vi "ep_Check Error (N CH).vi"(0 "spectra information":T1, 5 "slip":dbl[](array[numeric]), 7 "max sideband order (10)":u8=10, 9 "fundamental frequency [Hz]":dbl, 11 "error in (no error)":errorcluster) -> (4 "dup spectra information":T1, 6 "dup slip":dbl[](array[numeric]), 10 "dup fundamental frequency [Hz]":dbl, 15 "error out":errorcluster)   [LabVIEW 2014, in "NI_EP_Motor Monitoring.lvlib"]
uses:
  <vilib>/addons/Electrical Power/Motor Monitoring/NI_EP_Motor Monitoring.lvlib
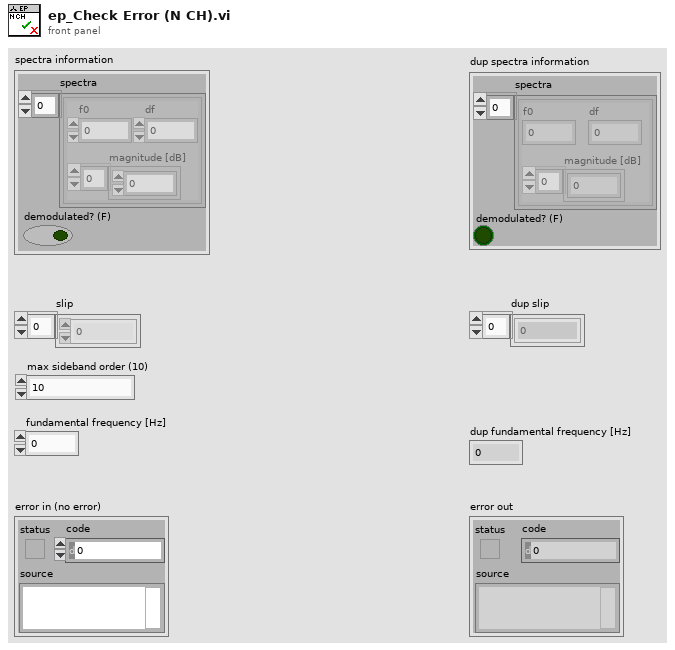
[diagram p1: front panel]
types:
  T1 = cluster{"spectra":cluster{"f0":dbl, "df":dbl, "magnitude [dB]":dbl[]}[], "demodulated? (F)":bool}
  T2 = cluster{"f0":dbl, "df":dbl, "magnitude [dB]":dbl[]}[]
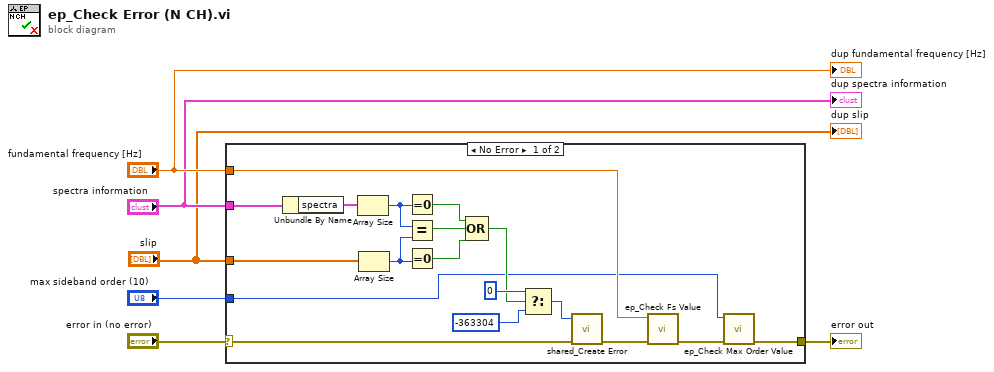
[diagram p0: block diagram]
diagram:
  n1 = case shown="No Error" "error in (no error)" {
    selector: "error in (no error)" -> [w19 w25]
    tunnel: "spectra information" -> [w21 _]
    tunnel: "slip" -> [w10 _]
    tunnel: "fundamental frequency [Hz]" -> [w11 _]
    tunnel: [w8 w25] -> w5
    tunnel: "max sideband order (10)" -> [w7 _]
    frame No Error {
      n2 = Unbundle By Name(w21) -> ("spectra"=w20:T2)
      n3 = Array Size(array=w20) -> (size(s)=w12:i32)
      n4 = Array Size(array=w10) -> (size(s)=w17:i32)
      n5 = Equal To 0?(x=w12) -> (x = 0?=w16:bool)
      n6 = Equal?(x=w12, y=w17) -> (x = y?=w15:bool)
      n7 = Equal To 0?(x=w17) -> (x = 0?=w14:bool)
      n8 = Compound Arithmetic op=OR(w16, w15, w14) -> (w13:bool)
      n9 = Select(t=0 ("error code (0)"), s=w13, f=-363304 ("error code (0)")) -> (s? t:f=w22:i32)
      n10 = call <vilib>:"shared_Create Error.vi"("error in (no error)"=w19, "error code (0)"=w22) -> ("error out"=w18:errorcluster)  [unwired: 9 in]
      n11 = call <vilib>:"ep_Check Fs Value.vi"("error in (no error)"=w18, "fundamental frequency [Hz]"=w11) -> ("error out"=w9:errorcluster)  [unwired: 9 in]
      n12 = call <vilib>:"ep_Check Max Order Value.vi"("error in (no error)"=w9, "max sideband order"=w7) -> ("error out"=w8:errorcluster)  [unwired: 9 in]
    }
    frame Error {
    }
  }
  "error out" <- w5
  "dup fundamental frequency [Hz]" <- "fundamental frequency [Hz]"
  "dup spectra information" <- "spectra information"
  "dup slip" <- "slip"
